vi "pionowy.vi"(4 "Akcja":T1, 5 "pauza":bool) -> (1 "Aktualny stan":T2, 2 "KONIEC":bool)   [LabVIEW 2014]
uses:
  main_states_2.ctl
  Akcje.ctl
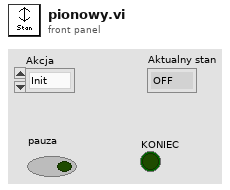
[diagram p1: front panel]
types:
  T1 = typedef "Akcje.ctl" = enum16{"Init", "Przygotuj listę", "Sprawdź"}
  T2 = typedef "main_states_2.ctl" = enum16{"OFF", "UP", "DOWN", "MANUAL"}
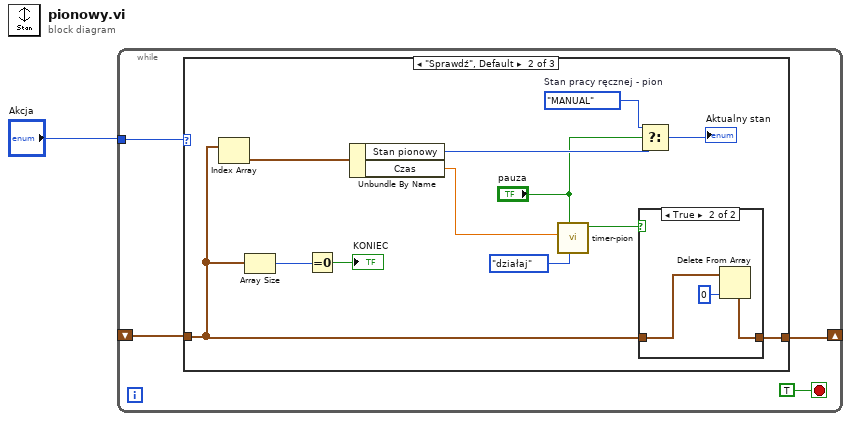
[diagram p0: block diagram]
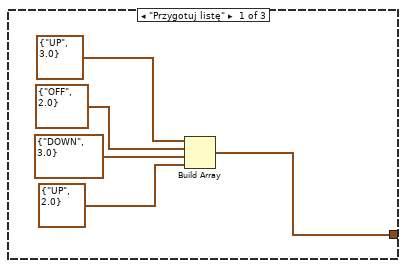
[diagram p2: hidden frame]
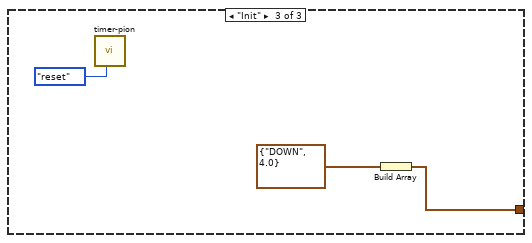
[diagram p4: hidden frame]
diagram:
  n1 = while {
    tunnel: "Akcja" -> [w4]
    shift-right: [w3] -> _
    shift-left: _ -> [w2]
    stop <- TRUE stop-if-true
    n2 = case shown="\"Sprawdź\", Default" w4 {
      tunnel: [w6 w22 w28] -> w3
      tunnel: w2 -> [_ w18 _]
      frame "Przygotuj listę" {
        n3 = Build Array(cluster{"Stan pionowy":T2, "Czas":dbl} {"Stan pionowy"=enum."UP", "Czas"=3.0} ("Cluster"), cluster{"Stan pionowy":T2, "Czas":dbl} {"Stan pionowy"=enum."OFF", "Czas"=2.0} ("Cluster"), cluster{"Stan pionowy":T2, "Czas":dbl} {"Stan pionowy"=enum."DOWN", "Czas"=3.0} ("Cluster"), cluster{"Stan pionowy":T2, "Czas":dbl} {"Stan pionowy"=enum."UP", "Czas"=2.0} ("Cluster")) -> (w6:cluster{"Stan pionowy":T2, "Czas":dbl}[])
      }
      frame "Sprawdź", Default {
        w20 = main_states_2."MANUAL"  # Stan pracy ręcznej - pion
        n4 = Index Array(array=w18) -> (element=w15:cluster{"Stan pionowy":T2, "Czas":dbl})  [unwired: 1 in]
        n5 = Array Size(array=w18) -> (size(s)=w17:i32)
        n6 = Equal To 0?(x=w17) -> (x = 0?=→"KONIEC":bool)
        n7 = Unbundle By Name(w15) -> ("Stan pionowy"=w21:T2, "Czas"=w14:dbl)
        n8 = call "timer-pion.vi"("Czynność"=enum16{"reset", "działaj"}."działaj", "pauza"="pauza", "Czas"=w14) -> ("czy czas upłynął"=w12:bool)  [unwired: 8 in]
        n9 = case shown="True" w12 {
          tunnel: [w23 w26] -> w22
          tunnel: w18 -> [w23 w24]
          frame False {
          }
          frame True {
            n10 = Delete From Array(array=w24, index=0) -> (array with subset deleted=w26:cluster{"Stan pionowy":T2, "Czas":dbl}[])  [unwired: 1 in, 1 out]
          }
        }
        n11 = Select(t=w20, s="pauza", f=w21) -> (s? t:f=→"Aktualny stan":T2)
      }
      frame "Init" {
        n12 = call "timer-pion.vi"("Czynność"=enum16{"reset", "działaj"}."reset") -> ()  [unwired: 10 in, 1 out]
        n13 = Build Array(cluster{"Stan pionowy":T2, "Czas":dbl} {"Stan pionowy"=enum."DOWN", "Czas"=4.0} ("Cluster")) -> (w28:cluster{"Stan pionowy":T2, "Czas":dbl}[])
      }
    }
  }
